vi "Test Gain.vi"(11 "Test Case In":refnum<class "Test.Camera.lvclass">) -> (0 "error out":errorcluster, 3 "Test Case Out":refnum<class "Test.Camera.lvclass">)   [LabVIEW 2020, in "Test.Camera.lvclass"]
uses:
  Test.Camera.lvclass
  C:/Program Files (x86)/National Instruments/LabVIEW 2020/vi.lib/Astemes/LUnit/Test Case.lvclass
  g_industrial_cam/Camera/Camera.lvclass/Camera.ctl
  <vilib>/Astemes/LUnit/Test Case.lvclass/Test Case.ctl
  c3e2611f-c54f-4219-a549-b8da21c7f085.vi
  9d545e64-2dc1-465e-bc57-1cc83b6d681a.vi
  bb3897f6-d6c9-4df8-9efa-d93feb0c7bd0.vi
  2762433e-4530-4928-a342-cb688c9c0257.vi
  9195b4cb-d389-4eeb-9708-177fb2e26729.vi
  g_industrial_cam/Camera/GetSetGain.vi
  g_industrial_cam/Camera/GetSetGainAuto.vi
  <vilib>/Astemes/LUnit/Core/LUnit Test Case/Private/Append Pass Result.vi
  <vilib>/Astemes/LUnit/Core/LUnit Test Case/Private/Append Fail Result.vi
  9d545e64-2dc1-465e-bc57-1cc83b6d681a.vi/23ce184e-9622-4817-bac2-1c972340de52.vi
  9d545e64-2dc1-465e-bc57-1cc83b6d681a.vi/3848369b-d3fa-48af-9fdc-8c3f580b91af.vi
  bb3897f6-d6c9-4df8-9efa-d93feb0c7bd0.vi/9c5d11cd-9439-4240-a1ee-d9baace9c924.vi
  9195b4cb-d389-4eeb-9708-177fb2e26729.vi/9c5d11cd-9439-4240-a1ee-d9baace9c924.vi
  <vilib>/Astemes/LUnit/Core/LUnit Test Case/Private/Run In UI.vi
  <vilib>/Utility/error.llb/Clear Errors.vi
  g_industrial_cam/Camera/Check Not Disconnected.vi
  <vilib>/Utility/error.llb/Error Cluster From Error Code.vi
  <vilib>/Comparison/Equal/Equal Functor/Equal Functor.lvclass
  Test.Camera.lvclass/Test.Camera.ctl
  <vilib>/Astemes/LUnit/Test Case.lvclass
  g_industrial_cam/Camera/Camera.lvclass
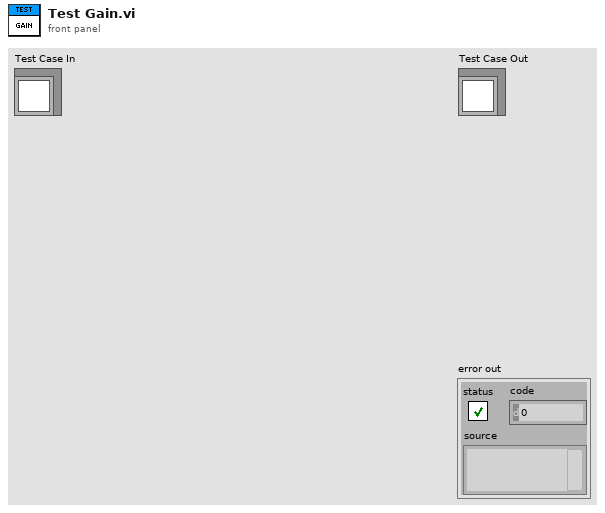
[diagram p1: front panel]
types:
  T1 = enum16{"Get Values", "Select Gain", "Set Auto", "Set Gain"}
  T2 = enum16{"Get Values", "Select Gain", "Set Auto", "Set Gain"}[]
  T3 = typedef "Camera.lvclass/Auto Mode.ctl" = enum8{"Off", "Once", "Continuous"}
  T4 = typedef "Camera.lvclass/Representation.ctl" = enum8{"Undefined", "Linear", "Logarithmic", "Boolean", "Pure Number", "Hex Number", "IP Address", "MAC Address"}
  T5 = cluster{"Avaliable":bool, "Representation":T4, "Min":dbl, "Max":dbl, "Mode":T3, "Auto Avaliable":bool, "Gain":dbl, "Available Gains":string[]}
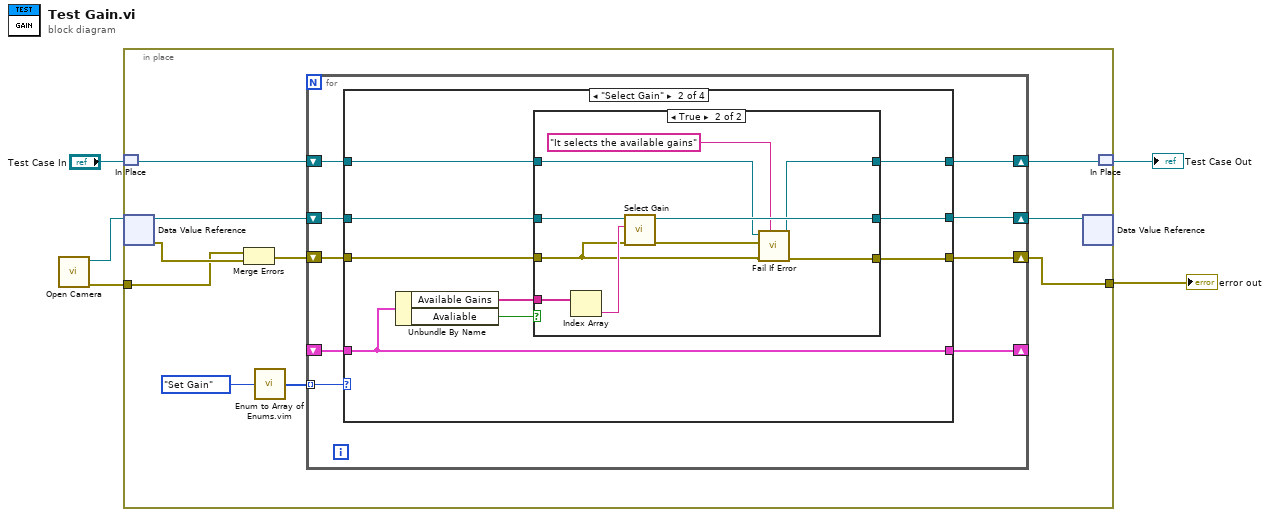
[diagram p0: block diagram]
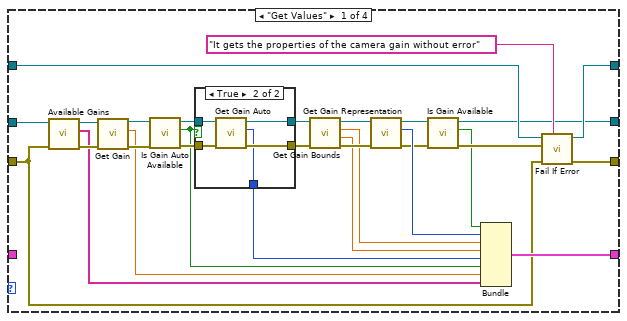
[diagram p2: hidden frame]
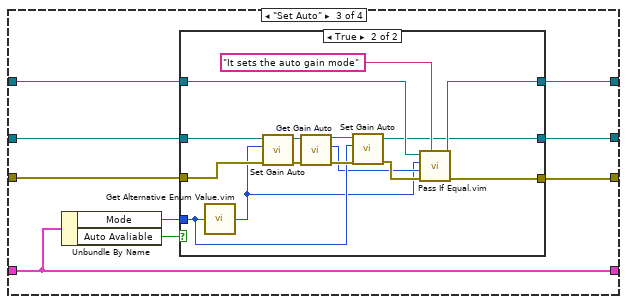
[diagram p5: hidden frame]
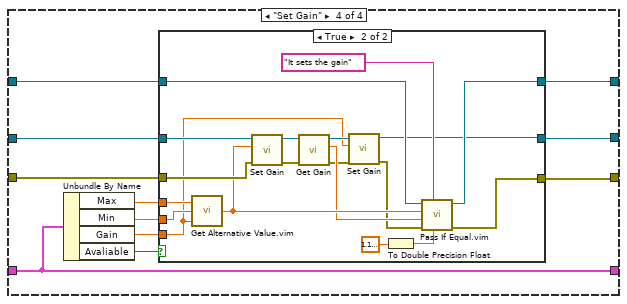
[diagram p7: hidden frame]
diagram:
  n1 = call "Open Camera.vi"() -> ("error out"=w5:errorcluster, "Camera"=w4:refnum<data-value>)  [unwired: 10 in]
  n2 = in-place {
    in-place-border: w5 -> [w7]
    in-place-border: [w6] -> w2
    n3 = in-place-match #1("Test Case In") -> (w10:refnum<class "Test.Camera.lvclass">)
    n4 = in-place-dvr #2(w4) -> (w14:refnum<class "Camera.lvclass">, w15:errorcluster)
    n5 = Merge Errors(w7, w15) -> (w13:errorcluster)
    n6 = call "Enum to Array of Enums.vim"("enum"=T1."Set Gain") -> ("array of enums"=w11:T2)
    n7 = for {
      tunnel: w11 -> [w22] mode=indexing
      shift-right: [w21] -> w8
      shift-left: w14 -> [w24]
      shift-right: [w20] -> _
      shift-left: _ -> [w19]
      shift-right: [w17] -> w9
      shift-left: w10 -> [w18]
      shift-right: [w16] -> w6
      shift-left: w13 -> [w23]
      n8 = case shown="\"Select Gain\"" w22 {
        tunnel: w24 -> [w53 w69 w91 w120]
        tunnel: w23 -> [w32 w66 w89 w118]
        tunnel: [w26 w64 w87 w116] -> w21
        tunnel: [w35 w68 w90 w119] -> w20
        tunnel: w19 -> [_ w68 w90 w119]
        tunnel: w18 -> [w34 w63 w86 w115]
        tunnel: [w33 w62 w85 w114] -> w17
        tunnel: [w29 w65 w88 w117] -> w16
        frame "Get Values" {
          n9 = call "Available Gains.vi"("error in (no error)"=w32, "Camera in"=w53) -> ("error out"=w50:errorcluster, "Available Gains"=w42:string[], "Camera"=w52:refnum<class "Camera.lvclass">)  [unwired: 7 in]
          n10 = call "Get Gain.vi"("error in (no error)"=w50, "Camera in"=w52) -> ("error out"=w49:errorcluster, "Gain"=w41:dbl, "Camera"=w51:refnum<class "Camera.lvclass">)  [unwired: 7 in]
          n11 = call "Is Gain Auto Available.vi"("error in (no error)"=w49, "Camera in"=w51) -> ("error out"=w48:errorcluster, "Auto Avaliable"=w40:bool, "Camera"=w47:refnum<class "Camera.lvclass">)  [unwired: 7 in]
          n12 = case shown="True" w40 {
            tunnel: w48 -> [w54 w60]
            tunnel: w47 -> [w55 w59]
            tunnel: [w55 w58] -> w45
            tunnel: [w54 w57] -> w46
            tunnel: [_ w56] -> w39
            frame False {
            }
            frame True {
              n13 = call "Get Gain Auto.vi"("error in (no error)"=w60, "Camera in"=w59) -> ("error out"=w57:errorcluster, "Mode"=w56:T3, "Camera"=w58:refnum<class "Camera.lvclass">)  [unwired: 7 in]
            }
          }
          n14 = call "Get Gain Bounds.vi"("error in (no error)"=w46, "Camera in"=w45) -> ("error out"=w44:errorcluster, "Max"=w38:dbl, "Min"=w37:dbl, "Camera"=w43:refnum<class "Camera.lvclass">)  [unwired: 6 in]
          n15 = call "Get Gain Representation.vi"("error in (no error)"=w44, "Camera in"=w43) -> ("error out"=w31:errorcluster, "Representation"=w36:T4, "Camera"=w27:refnum<class "Camera.lvclass">)  [unwired: 7 in]
          n16 = call "Is Gain Available.vi"("error in (no error)"=w31, "Camera in"=w27) -> ("error out"=w28:errorcluster, "Avaliable"=w25:bool, "Camera"=w26:refnum<class "Camera.lvclass">)  [unwired: 7 in]
          n17 = Bundle("Avaliable"=w25, "Representation"=w36, "Min"=w37, "Max"=w38, "Mode"=w39, "Auto Avaliable"=w40, "Gain"=w41, "Available Gains"=w42) -> (w35:T5)  [unwired: 1 in]
          n18 = call <vilib>:"Fail If Error.vi"("Description"="It gets the properties of the camera gain without error", "error in (no error)"=w32, "Assert error"=w28, "LUnit Test Case In"=w34) -> ("error out"=w29:errorcluster, "LUnit Test Case Out"=w33:refnum<class "Test.Camera.lvclass">)  [unwired: 6 in]
        }
        frame "Select Gain" {
          n19 = Unbundle By Name(w68) -> ("Available Gains"=w67:string[], "Avaliable"=w61:bool)
          n20 = case shown="True" w61 {
            tunnel: w69 -> [w72 w82]
            tunnel: w67 -> [_ w81]
            tunnel: w66 -> [w71 w78]
            tunnel: [w71 w77] -> w65
            tunnel: [w72 w76] -> w64
            tunnel: w63 -> [w70 w75]
            tunnel: [w70 w74] -> w62
            frame False {
            }
            frame True {
              n21 = Index Array(array=w81) -> (element=w80:string)  [unwired: 1 in]
              n22 = call "Select Gain.vi"("error in (no error)"=w78, "Selection"=w80, "Camera in"=w82) -> ("error out"=w79:errorcluster, "Camera"=w76:refnum<class "Camera.lvclass">)  [unwired: 7 in]
              n23 = call <vilib>:"Fail If Error.vi"("Description"="It selects the available gains", "error in (no error)"=w78, "Assert error"=w79, "LUnit Test Case In"=w75) -> ("error out"=w77:errorcluster, "LUnit Test Case Out"=w74:refnum<class "Test.Camera.lvclass">)  [unwired: 6 in]
            }
          }
        }
        frame "Set Auto" {
          n24 = Unbundle By Name(w90) -> ("Mode"=w83:T3, "Auto Avaliable"=w84:bool)
          n25 = case shown="True" w84 {
            tunnel: w91 -> [w94 w109]
            tunnel: w89 -> [w93 w107]
            tunnel: [w93 w106] -> w88
            tunnel: [w94 w97] -> w87
            tunnel: w86 -> [w92 w105]
            tunnel: [w92 w104] -> w85
            tunnel: w83 -> [_ w98]
            frame False {
            }
            frame True {
              n26 = call "Get Alternative Enum Value.vim"("Enum In"=w98) -> ("Alternative Value"=w95:T3)
              n27 = call "Set Gain Auto.vi"("error in (no error)"=w107, "Mode"=w95, "Camera in"=w109) -> ("error out"=w108:errorcluster, "Camera"=w102:refnum<class "Camera.lvclass">)  [unwired: 7 in]
              n28 = call "Get Gain Auto.vi"("error in (no error)"=w108, "Camera in"=w102) -> ("error out"=w101:errorcluster, "Mode"=w96:T3, "Camera"=w100:refnum<class "Camera.lvclass">)  [unwired: 7 in]
              n29 = call "Set Gain Auto.vi"("error in (no error)"=w101, "Mode"=w98, "Camera in"=w100) -> ("error out"=w99:errorcluster, "Camera"=w97:refnum<class "Camera.lvclass">)  [unwired: 7 in]
              n30 = call "Pass If Equal.vim"("Description"="It sets the auto gain mode", "error in (no error)"=w99, "Actual"=w96, "Expected"=w95, "LUnit Test Case In"=w105) -> ("error out"=w106:errorcluster, "LUnit Test Case Out"=w104:refnum<class "Test.Camera.lvclass">)  [unwired: 5 in]
            }
          }
        }
        frame "Set Gain" {
          n31 = Unbundle By Name(w119) -> ("Max"=w112:dbl, "Min"=w111:dbl, "Gain"=w110:dbl, "Avaliable"=w113:bool)
          n32 = case shown="True" w113 {
            tunnel: w120 -> [w123 w136]
            tunnel: w118 -> [w122 w133]
            tunnel: [w122 w142] -> w117
            tunnel: [w123 w127] -> w116
            tunnel: w115 -> [w121 w141]
            tunnel: [w121 w140] -> w114
            tunnel: w112 -> [_ w138]
            tunnel: w111 -> [_ w137]
            tunnel: w110 -> [_ w128]
            frame False {
            }
            frame True {
              n33 = call "Get Alternative Value.vim"("Value"=w128, "Min"=w137, "Max"=w138) -> ("Alternative Value"=w132:dbl)  [unwired: 1 in]
              n34 = call "Set Gain.vi"("error in (no error)"=w133, "Gain"=w132, "Camera in"=w136) -> ("error out"=w134:errorcluster, "Camera"=w135:refnum<class "Camera.lvclass">)  [unwired: 7 in]
              n35 = call "Get Gain.vi"("error in (no error)"=w134, "Camera in"=w135) -> ("error out"=w129:errorcluster, "Gain"=w131:dbl, "Camera"=w130:refnum<class "Camera.lvclass">)  [unwired: 7 in]
              n36 = call "Set Gain.vi"("error in (no error)"=w129, "Gain"=w128, "Camera in"=w130) -> ("error out"=w126:errorcluster, "Camera"=w127:refnum<class "Camera.lvclass">)  [unwired: 7 in]
              n37 = To Double Precision Float(number=sgl 1.1920929e-07) -> (double precision float=w124:dbl)
              n38 = call "Pass If Equal.vim"("Delta"=w124, "Description"="It sets the gain", "error in (no error)"=w126, "Actual"=w131, "Expected"=w132, "LUnit Test Case In"=w141) -> ("error out"=w142:errorcluster, "LUnit Test Case Out"=w140:refnum<class "Test.Camera.lvclass">)  [unwired: 4 in]
            }
          }
        }
      }
    }
    n39 = in-place-dvr #2(w8) -> ()  [unwired: 2 out]
    n40 = in-place-match #1(w9) -> (→"Test Case Out":refnum<class "Test.Camera.lvclass">)
  }
  "error out" <- w2
